vi "Get SMO Name.vi"(8 "error in (no error)":errorcluster, 11 "Sequence Experiment":refnum<class "Control Experiment.lvclass">) -> (0 "error out":errorcluster, 2 "SMO Name":string, 3 "Sequence Experiment out":refnum<class "Control Experiment.lvclass">)   [LabVIEW 2016, in "Control Experiment.lvclass"]
uses:
  Control Experiment.lvclass
  <userlib>/LevyLab/Levylab Instruments/SMOs/Instrument/Instrument.lvclass
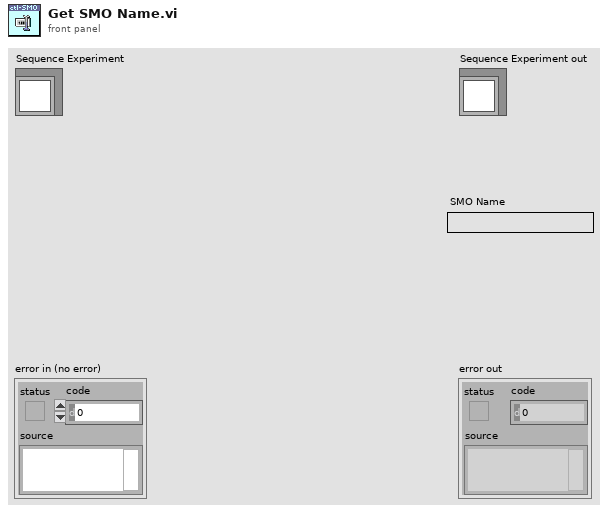
[diagram p1: front panel]
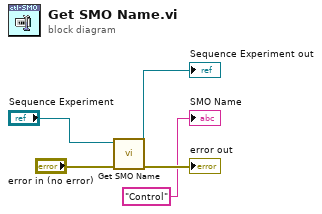
[diagram p0: block diagram]
diagram:
  n1 = call-parent "Get SMO Name.vi"("error in (no error)"="error in (no error)", "Instrument in"="Sequence Experiment") -> ("error out"=→"error out":errorcluster, "Instrument out"=→"Sequence Experiment out":refnum<class "Control Experiment.lvclass">)  [unwired: 7 in, 1 out]
  "SMO Name" <- "Control" ("SMO Name")
